vi "Fix Coloring Offset.vi"(8 "error in (no error)":errorcluster, 9 "# LB Tests":i32, 10 "TopLevel":T1) -> (0 "error out":errorcluster)   [LabVIEW 2011]
uses:
  Controls/Top Level Control.ctl
  <vilib>/NI/AMC/Message Queue.ctl
  <vilib>/NI/AMC/Message.ctl
  <vilib>/NI/Tools/Keyed Array/KeyedArray.ctl
  Controls/ListBox Test Record.ctl
  Controls/DVR of CSV Tests Data.ctl
  Controls/CSVs Tests Data.ctl
  Controls/Test Column Data.ctl
  Controls/Options DVR.ctl
  Controls/Options.ctl
  <vilib>/NI/Tools/Keyed Array/Tools_KeyedArray.lvlib
  <vilib>/NI/AMC/AMC.lvlib
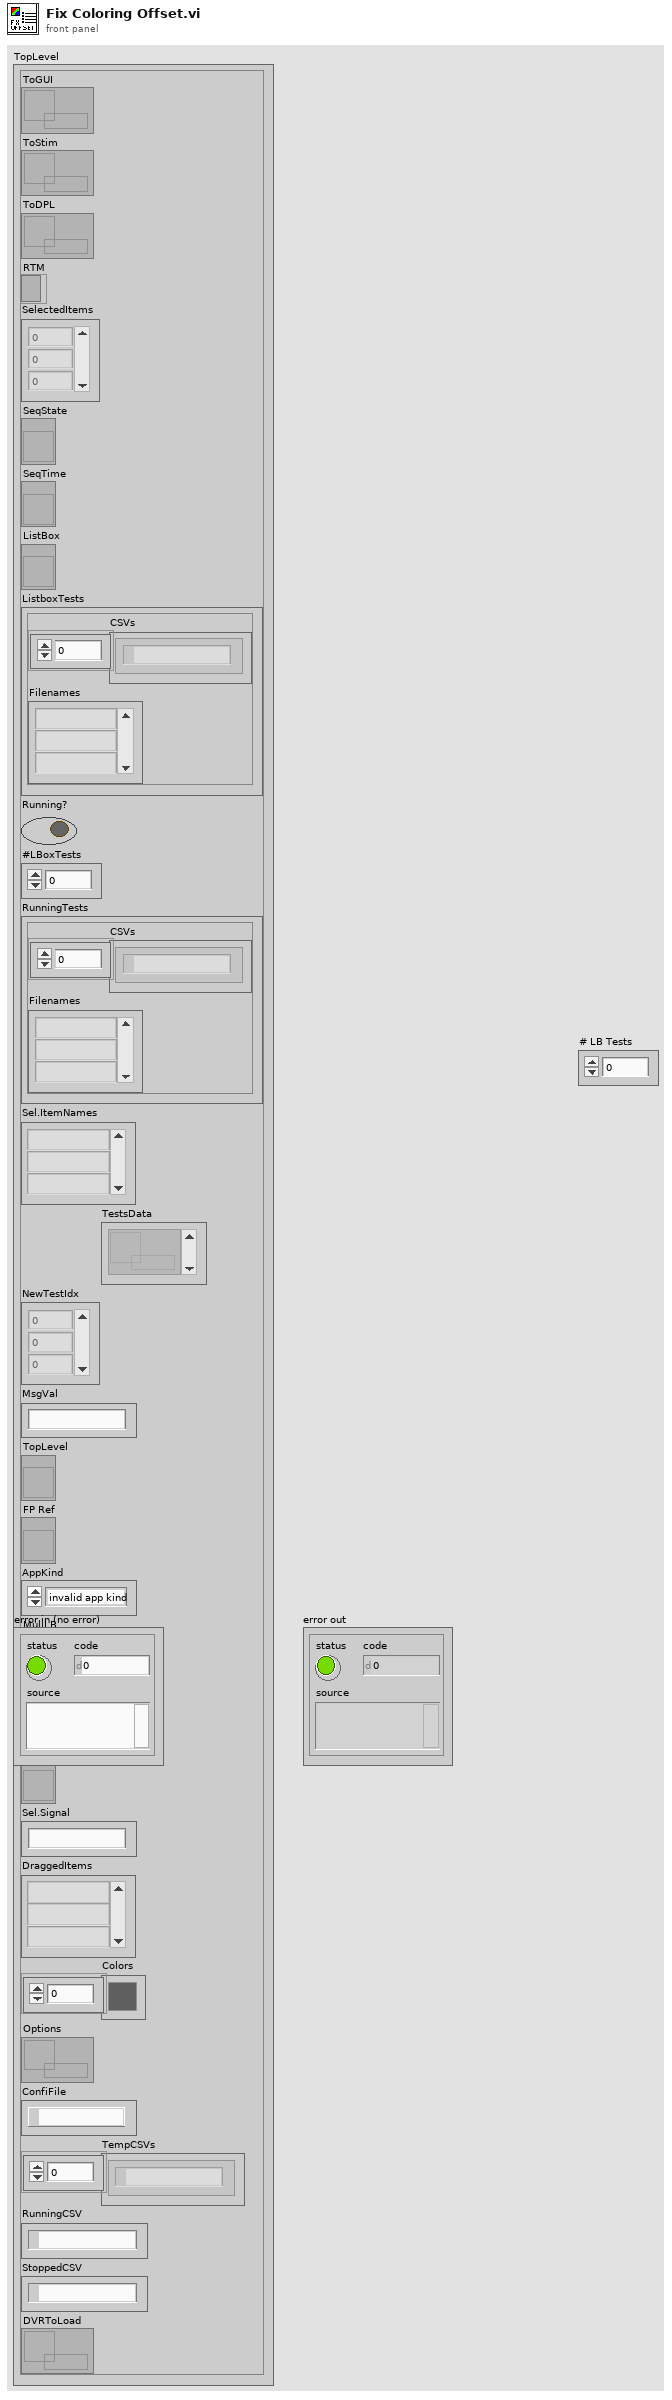
[diagram p1: front panel]
types:
  T1 = typedef "Top Level Control.ctl" = cluster{"ToGUI":T2, "ToStim":T2, "ToDPL":T2, "RTM":refnum<k9>, "SelectedItems":i32[], "SeqState":refnum<vi>, "SeqTime":refnum<vi>, "ListBox":refnum<vi>, "ListboxTests":T3, "Running?":bool, "#LBoxTests":i32, "RunningTests":T3, "Sel.ItemNames":string[], "TestsData":T4[], "NewTestIdx":i32[], "MsgVal":string, "TopLevel":refnum<vi>, "FP Ref":refnum<vi>, "AppKind":enum32{"invalid app kind", "Development System", "Run Time System", "Student Edition", "Embedded LabVIEW", "Evaluation", "Custom"}, "MuliLB":refnum<vi>, "Ring":refnum<vi>, "Graph":refnum<vi>, "Sel.Signal":string, "DraggedItems":string[], "Colors":u32[], "Options":T5, "ConfiFile":path, "TempCSVs":path[], "RunningCSV":path, "StoppedCSV":path, "DVRToLoad":T4}
  T2 = typedef "AMC.lvlib/Message Queue.ctl" = refnum<queue>
  T3 = typedef "ListBox Test Record.ctl" = cluster{"CSVs":path[], "Filenames":string[]}
  T4 = typedef "DVR of CSV Tests Data.ctl" = refnum<data-value>
  T5 = typedef "Options DVR.ctl" = refnum<data-value>
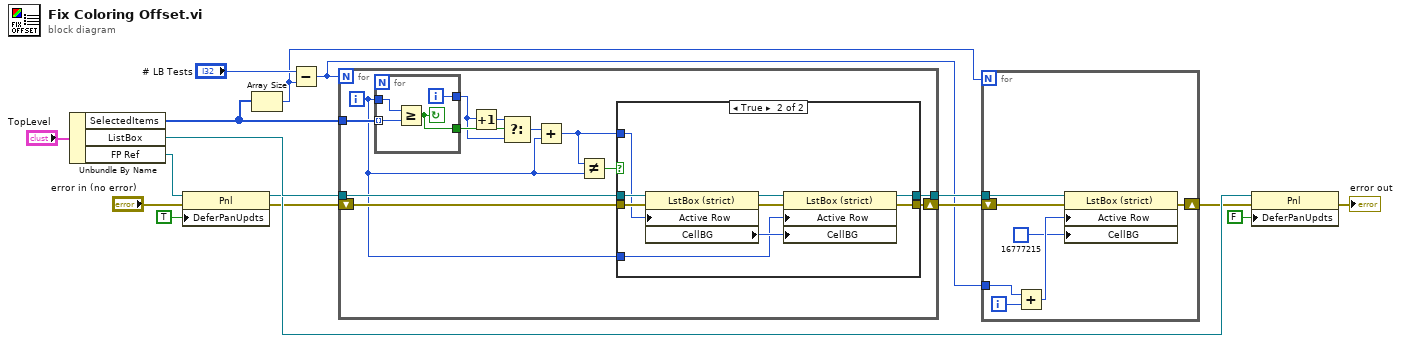
[diagram p0: block diagram]
diagram:
  n1 = Unbundle By Name("TopLevel") -> ("SelectedItems"=w7:i32[], "ListBox"=w16:refnum<vi>, "FP Ref"=w14:refnum<vi>)
  n2 = property on="Property Node" class="Pnl"(reference=w14, error in="error in (no error)", "DeferPanUpdts"=TRUE ("Defer Panel Updates")) -> (reference out=w11:refnum<vi>, error out=w10:errorcluster)
  n3 = Array Size(array=w7) -> (size(s)=w4:i32)
  n4 = Subtract(x="# LB Tests", y=w4) -> (x-y=w1:i32)
  n5 = for {
    N: w1 -> [_]
    tunnel: w16 -> [w27]
    shift-right: [w28] -> w5
    shift-left: w10 -> [w26]
    tunnel: w7 -> [w25]
    tunnel: [w19] -> w3
    i -> [w17]
    n6 = for {
      tunnel: w25 -> [w43] mode=indexing
      tunnel: w17 -> [w42]
      tunnel: [w41] -> w20
      tunnel: [w40] -> w23
      i -> [w41]
      stop <- w40 continue-if-true
      n7 = Greater Or Equal?(x=w42, y=w43) -> (x >= y?=w40:bool)
    }
    n8 = Increment(x=w20) -> (x+1=w22:i32)
    n9 = Select(t=w22, s=w23, f=w20) -> (s? t:f=w21:i32)
    n10 = Add(x=w21, y=w17) -> (x+y=w18:i32)
    n11 = Not Equal?(x=w18, y=w17) -> (x != y?=w24:bool)
    n12 = case shown="True" w24 {
      tunnel: [w30 w33] -> w28
      tunnel: w27 -> [w29 w39]
      tunnel: w26 -> [w30 w38]
      tunnel: w18 -> [_ w37]
      tunnel: w17 -> [_ w32]
      tunnel: [w29 w31] -> w19
      frame False {
      }
      frame True {
        n13 = property on="Property Node" class="LstBox (strict)"(reference=w39, error in=w38, "Active Row"=w37) -> (reference out=w36:refnum<vi>, error out=w35:errorcluster, "CellBG"=w34:u32)
        n14 = property on="Property Node" class="LstBox (strict)"(reference=w36, error in=w35, "Active Row"=w32, "CellBG"=w34) -> (reference out=w31:refnum<vi>, error out=w33:errorcluster)
      }
    }
  }
  n15 = for {
    N: w4 -> [_]
    shift-right: [w50] -> w2
    shift-left: w5 -> [w49]
    tunnel: w3 -> [w48]
    tunnel: w1 -> [w46]
    i -> [w47]
    n16 = Add(x=w46, y=w47) -> (x+y=w45:i32)
    n17 = property on="Property Node" class="LstBox (strict)"(reference=w48, error in=w49, "Active Row"=w45, "CellBG"=u32 16777215) -> (error out=w50:errorcluster)  [unwired: 1 out]
  }
  n18 = property on="Property Node" class="Pnl"(reference=w11, error in=w2, "DeferPanUpdts"=FALSE ("Defer Panel Updates")) -> (error out=→"error out":errorcluster)  [unwired: 1 out]
